vi "Scheduler.Core.vi"(8 "Error In":errorcluster, 9 "Data":variant, 10 "Cmd":string, 11 "Parent Q":refnum<queue>) -> (0 "Error Out":errorcluster, 1 "Exit":bool, 2 "Remaining ms":i32, 3 "Parent Q Out":refnum<queue>)   [LabVIEW 2024, in "EQMF.lvlib" / "Scheduler.lvlib"]
uses:
  Scheduler.lvlib
  Queues/Q.Element.ctl
  _Private/Scheduler.Item.ctl
  Queues/Queue Utils.lvlib
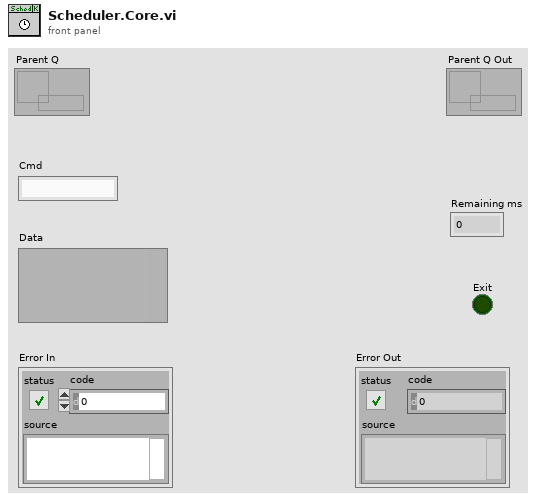
[diagram p1: front panel]
types:
  T1 = typedef "EQMF.lvlib/Scheduler.lvlib/Scheduler.Item.ctl" = cluster{"Name":string, "Start Time(s)":dbl, "Interval(s)":dbl, "Recurring":bool, "Q In":refnum<queue>, "Q.Element":T2}
  T2 = typedef "EQMF.lvlib/Queue Utils.lvlib/Q.Element.ctl" = cluster{"Cmd":string, "Sub":string, "Data1":variant, "Data2":variant}
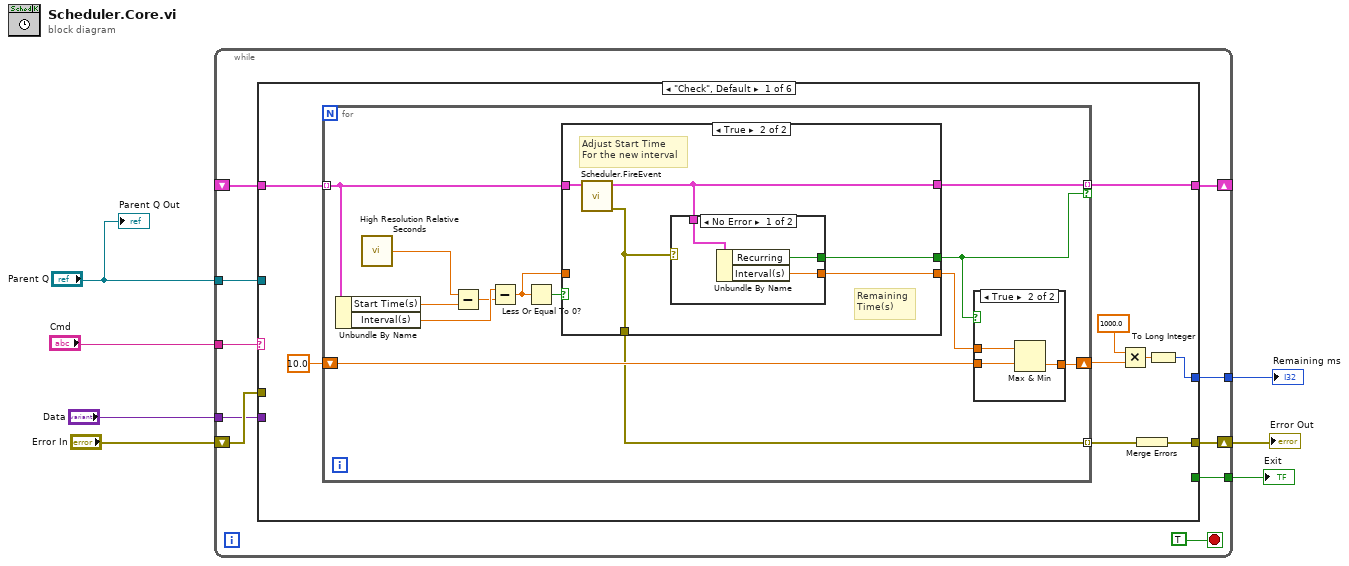
[diagram p0: block diagram]
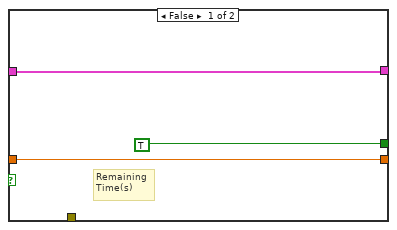
[diagram p3: hidden frame]
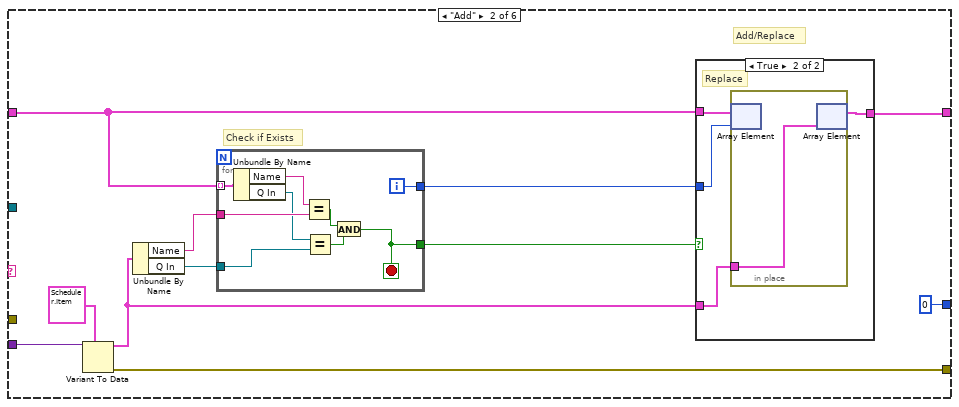
[diagram p5: hidden frame]
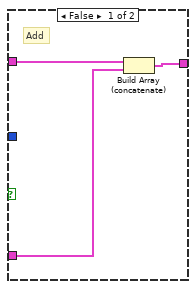
[diagram p6: hidden frame]
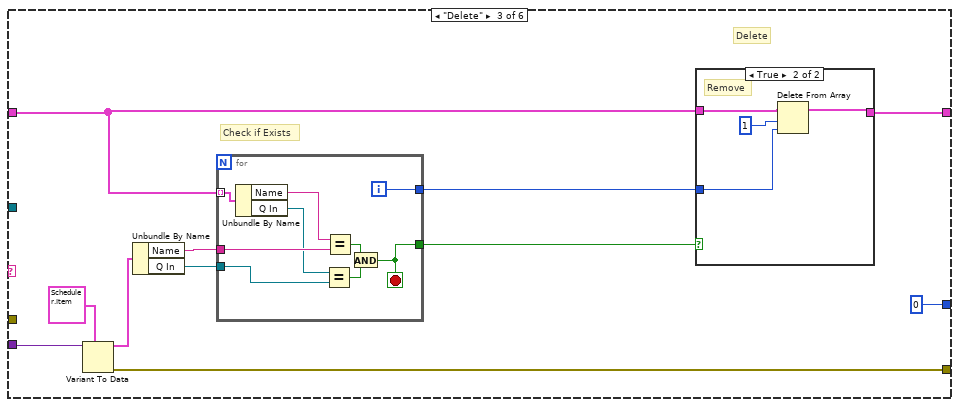
[diagram p7: hidden frame]
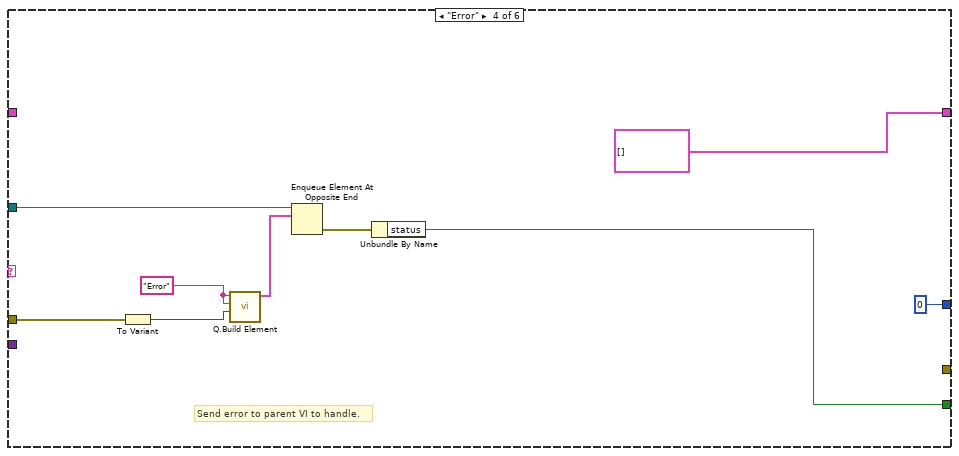
[diagram p9: hidden frame]
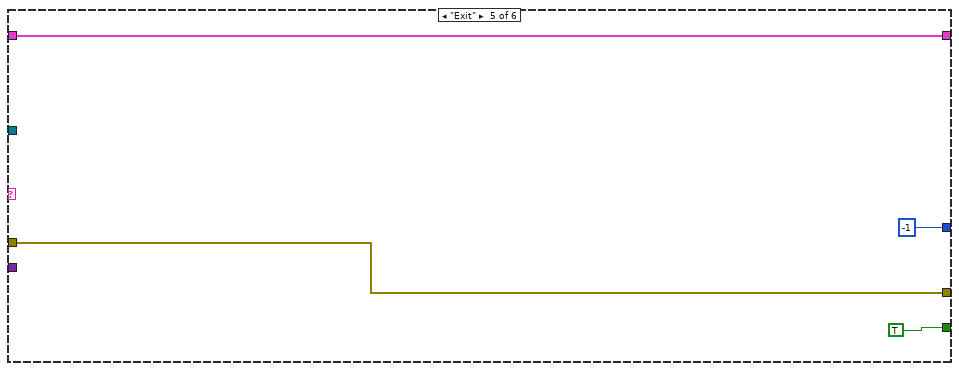
[diagram p10: hidden frame]
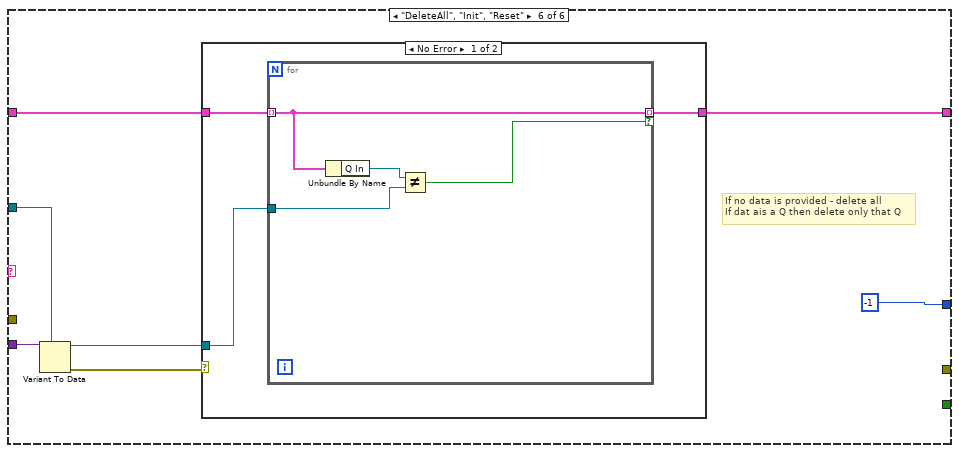
[diagram p11: hidden frame]
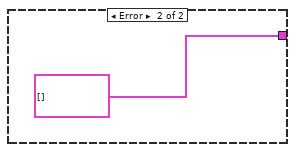
[diagram p12: hidden frame]
diagram:
  n1 = while {
    tunnel: "Parent Q" -> [w16]
    tunnel: "Cmd" -> [w15]
    tunnel: "Data" -> [w13]
    shift-right: [w12] -> w4
    shift-left: "Error In" -> [w14]
    tunnel: [w11] -> w2
    shift-right: [w9] -> _
    shift-left: _ -> [w17]
    tunnel: [w8] -> w1
    stop <- TRUE stop-if-true
    n2 = case shown="\"Check\", Default" w15 {
      tunnel: w13 -> [_ w57 w84 _ _ w125]
      tunnel: w14 -> [_ _ _ w115 w117 _]
      tunnel: w16 -> [_ _ _ w116 _ w124]
      tunnel: w17 -> [w26 w64 w92 _ w119 w122]
      tunnel: [w22 0 0 0 -1 -1] -> w11
      tunnel: [_ _ _ w108 TRUE _] -> w8
      tunnel: [w25 w60 w88 T1[] [] w119 w127] -> w9
      tunnel: [w19 w58 w85 _ w117 _] -> w12
      frame "Check", Default {
        n3 = for {
          tunnel: w26 -> [w37] mode=indexing
          tunnel: [w36] -> w25 mode=indexing if=w30
          shift-right: [w34] -> w20
          shift-left: 10.0 -> [w29]
          tunnel: [w28] -> w18 mode=indexing
          n4 = Unbundle By Name(w37) -> ("Start Time(s)"=w38:dbl, "Interval(s)"=w31:dbl)
          n5 = call <vilib>:"High Resolution Relative Seconds.vi"() -> ("relative seconds"=w39:dbl)
          n6 = Subtract(x=w39, y=w38) -> (x-y=w27:dbl)
          n7 = Subtract(x=w31, y=w27) -> (x-y=w32:dbl)
          n8 = Less Or Equal To 0?(x=w32) -> (x <= 0?=w33:bool)
          n9 = case shown="True" w33 {
            tunnel: w37 -> [w46 w51]
            tunnel: [w46 w48] -> w36
            tunnel: w32 -> [w44 _]
            tunnel: [TRUE w50] -> w30
            tunnel: [w44 w49] -> w35
            tunnel: [_ w47] -> w28
            frame False {
              # "Remaining\nTime(s)"
            }
            frame True {
              # "Adjust Start Time\nFor the new interval"
              # "Remaining\nTime(s)"
              n10 = call "Scheduler.FireEvent.vi"("Sched Item"=w51) -> ("error out"=w47:errorcluster, "Sched Item Out"=w48:T1)  [unwired: 9 in]
              n11 = case shown="No Error" w47 {
                tunnel: [w54 _] -> w50
                tunnel: [w53 _] -> w49
                tunnel: w48 -> [w52 _]
                frame No Error {
                  n12 = Unbundle By Name(w52) -> ("Recurring"=w54:bool, "Interval(s)"=w53:dbl)
                }
                frame Error {
                }
              }
            }
          }
          n13 = case shown="True" w30 {
            tunnel: w35 -> [_ w43]
            tunnel: [w40 w42] -> w34
            tunnel: w29 -> [w40 w41]
            frame False {
            }
            frame True {
              n14 = Max & Min(x=w43, y=w41) -> (min(x,y)=w42:dbl)  [unwired: 1 out]
            }
          }
        }
        n15 = Multiply(x=1000.0 ("y"), y=w20) -> (x*y=w23:dbl)
        n16 = Merge Errors(w18) -> (w19:errorcluster)
        n17 = To Long Integer(number=w23) -> (32bit integer=w22:i32)
      }
      frame "Add" {
        # "Add/Replace"
        # "Check if Exists"
        n18 = Variant To Data(type=T1 {"Name"="", "Start Time(s)"=0.0, "Interval(s)"=0.0, "Recurring"=FALSE, "Q In"=refnum, "Q.Element"={"Cmd"="", "Sub"="", "Data1"=variant, "Data2"=variant}}, Variant=w57) -> (data=w59:T1, error out=w58:errorcluster)  [unwired: 1 in]
        n19 = Unbundle By Name(w59) -> ("Name"=w65:string, "Q In"=w55:refnum<queue>)
        n20 = for {
          tunnel: w65 -> [w80]
          tunnel: w64 -> [w82] mode=indexing
          tunnel: [w74] -> w63
          tunnel: [w79] -> w62
          tunnel: w55 -> [w78]
          i -> [w79]
          stop <- w74 stop-if-true
          n21 = Unbundle By Name(w82) -> ("Name"=w81:string, "Q In"=w77:refnum<queue>)
          n22 = Equal?(x=w81, y=w80) -> (x = y?=w75:bool)
          n23 = Equal?(x=w77, y=w78) -> (x = y?=w76:bool)
          n24 = And(x=w75, y=w76) -> (x .and. y?=w74:bool)
        }
        n25 = case shown="True" w63 {
          tunnel: w64 -> [w68 w72]
          tunnel: w62 -> [_ w71]
          tunnel: w59 -> [w67 w70]
          tunnel: [w66 w69] -> w60
          frame False {
            # "Add"
            n26 = Build Array (concatenate)(w68, w67) -> (w66:T1[])
          }
          frame True {
            # "Replace"
            n27 = in-place {
              in-place-border: w70 -> [w73]
              n28 = in-place-array #1(w72, w71) -> ()  [unwired: 1 out]
              n29 = in-place-array #1(w73) -> (w69:T1[])  [unwired: 1 out]
            }
          }
        }
      }
      frame "Delete" {
        # "Delete"
        # "Check if Exists"
        n30 = Variant To Data(type=T1 {"Name"="", "Start Time(s)"=0.0, "Interval(s)"=0.0, "Recurring"=FALSE, "Q In"=refnum, "Q.Element"={"Cmd"="", "Sub"="", "Data1"=variant, "Data2"=variant}}, Variant=w84) -> (data=w87:T1, error out=w85:errorcluster)  [unwired: 1 in]
        n31 = Unbundle By Name(w87) -> ("Name"=w93:string, "Q In"=w83:refnum<queue>)
        n32 = for {
          tunnel: w93 -> [w105]
          tunnel: w92 -> [w107] mode=indexing
          tunnel: [w99] -> w91
          tunnel: [w104] -> w90
          tunnel: w83 -> [w102]
          i -> [w104]
          stop <- w99 stop-if-true
          n33 = Unbundle By Name(w107) -> ("Name"=w106:string, "Q In"=w103:refnum<queue>)
          n34 = Equal?(x=w103, y=w102) -> (x = y?=w101:bool)
          n35 = Equal?(x=w106, y=w105) -> (x = y?=w100:bool)
          n36 = And(x=w100, y=w101) -> (x .and. y?=w99:bool)
        }
        n37 = case shown="True" w91 {
          tunnel: w92 -> [w94 w98]
          tunnel: w90 -> [_ w97]
          tunnel: [w94 w95] -> w88
          frame False {
            # "Do Nothing"
          }
          frame True {
            # "Remove"
            n38 = Delete From Array(array=w98, length=1, index=w97) -> (array with subset deleted=w95:T1[])  [unwired: 1 out]
          }
        }
      }
      frame "Error" {
        w112 = "Error" ("Cmd")
        # "Send error to parent VI to handle."
        n39 = To Variant(anything=w115) -> (Variant=w111:variant)
        n40 = call "Q.Build Element.vi"("Data1"=w111, "Sub"=w112, "Cmd"=w112) -> ("Q.Element"=w110:T2)  [unwired: 8 in]
        n41 = Enqueue Element At Opposite End(queue=w116, element=w110) -> (error out=w109:errorcluster)  [unwired: 2 in, 2 out]
        n42 = Unbundle By Name(w109) -> ("status"=w108:bool)
      }
      frame "Exit" {
      }
      frame "DeleteAll", "Init", "Reset" {
        # "If no data is provided - delete all\nIf dat ais a Q then delete only that Q"
        n43 = Variant To Data(type=w124, Variant=w125) -> (data=w121:refnum<queue>, error out=w123:errorcluster)  [unwired: 1 in]
        n44 = case shown="No Error" w123 {
          tunnel: [w128 T1[] []] -> w127
          tunnel: w122 -> [w130 _]
          tunnel: w121 -> [w129 _]
          frame No Error {
            n45 = for {
              tunnel: w130 -> [w134] mode=indexing
              tunnel: w129 -> [w132]
              tunnel: [w134] -> w128 mode=indexing if=w131
              n46 = Unbundle By Name(w134) -> ("Q In"=w133:refnum<queue>)
              n47 = Not Equal?(x=w133, y=w132) -> (x != y?=w131:bool)
            }
          }
          frame Error {
          }
        }
      }
    }
  }
  "Error Out" <- w4
  "Remaining ms" <- w2
  "Exit" <- w1
  "Parent Q Out" <- "Parent Q"
